vi "15_25_Fxp_addation.vi"(1 "y":fxp<+/-,25,15>, 2 "x":fxp<+/-,25,15>) -> (0 "x+y":fxp<+/-,26,16> format="%.41g")   [LabVIEW 2020]
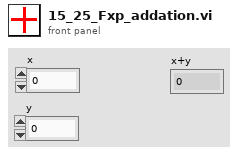
[diagram p1: front panel]
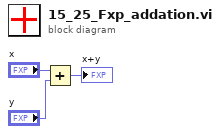
[diagram p0: block diagram]
diagram:
  n1 = Add(x="x", y="y") -> (x+y=→"x+y":fxp<+/-,26,16>)
